vi "Remove_FF_lone_spikes.vi"(5 "Analysis Info cluster In":T1={"Colour"=0, "Inst type"=enum."Pitot-static tube", "Inst name"="Manometer voltage", "Symbol"="U", "Code name"="", "Extra Info"="U", "Inst Array"=enum."PWA", "U"=0.0, "u^2"=0.0, "u^3"=0.0, "u^4"=0.0, "Skew_u"=0.0, "Kurt_u"=0.0, "Sd Error in Mean"=0.0, "% u'/U"=0.0, "X"=0.0, "Y"=0.0, "Z"=0.0, "Timescale integral Estimate"=0.0, "Sd Error in Variance"=0.0, "Calib File"=path "", "Calib Constants"=[], "Output Position"=FALSE, "Stats"=enum."None", "Av Sampling Rate"=0.0, "Av No of Samples"=0.0, "Total Meas Time (s)"=0.0, "OrigChName"="", "Max value"=0.0, "Min value"=0.0, "Req Sample Rate Hz"=0.0, "Sync Delay Time (s)"=0.0, "Ch No"=0, "Device"="", "Use Latest Calib"=FALSE, "Port"="", "Metadata Ch Names"=[], "Metadata Ch Values"=[], "Label"="", "chState"=enum."Solo", "Point Drift"=0.0, "inputConfig"=""} {"Kurt_u" format="%_3g"; "u^4" format="%_3g"; "u^3" format="%_3g"; "Sd Error in Variance" format="%_3g"; "u^2" format="%_3g"; "Sd Error in Mean" format="%_3g"; "U" format="%_3g"; "Sync Delay Time (s)" format="%.4f"; "Total Meas Time (s)" format="%_5g"; "Skew_u" format="%_3g"; "% u'/U" format="%_3g"}, 6 "Average Sampling Rate":dbl, 7 "index of element":i32, 8 "Per Block Plug Ins":string[](array[string]), 9 "Time Trace":dbl[](array[numeric])) -> (3 "Filtered Time Trace":dbl[](array[numeric]), 4 "Analysis Info cluster Out":T1={"Colour"=0, "Inst type"=enum."Pitot-static tube", "Inst name"="Manometer voltage", "Symbol"="U", "Code name"="", "Extra Info"="U", "Inst Array"=enum."PWA", "U"=0.0, "u^2"=0.0, "u^3"=0.0, "u^4"=0.0, "Skew_u"=0.0, "Kurt_u"=0.0, "Sd Error in Mean"=0.0, "% u'/U"=0.0, "X"=0.0, "Y"=0.0, "Z"=0.0, "Timescale integral Estimate"=0.0, "Sd Error in Variance"=0.0, "Calib File"=path "", "Calib Constants"=[], "Output Position"=FALSE, "Stats"=enum."None", "Av Sampling Rate"=0.0, "Av No of Samples"=0.0, "Total Meas Time (s)"=0.0, "OrigChName"="", "Max value"=0.0, "Min value"=0.0, "Req Sample Rate Hz"=0.0, "Sync Delay Time (s)"=0.0, "Ch No"=0, "Device"="", "Use Latest Calib"=FALSE, "Port"="", "Metadata Ch Names"=[], "Metadata Ch Values"=[], "Label"="", "chState"=enum."Solo", "Point Drift"=0.0, "inputConfig"=""} {"Kurt_u" format="%_3g"; "u^4" format="%_3g"; "u^3" format="%_3g"; "Sd Error in Variance" format="%_3g"; "u^2" format="%_3g"; "Sd Error in Mean" format="%_3g"; "U" format="%_3g"; "Sync Delay Time (s)" format="%.4f"; "Total Meas Time (s)" format="%_5g"; "Skew_u" format="%_3g"; "% u'/U" format="%_3g"})   [LabVIEW 2022 SP3]
uses:
  Globals/Meas_global.vi
  Controls/Inst_type.ctl
  Controls/Instrument_Array.ctl
  Controls/Analysis_info_cluster.ctl
  Controls/channelState.ctl
panel:
  out "Spikes Array Out":cluster{"Index":i32, "max value":dbl}[](array[cluster])
  out "Spikes Removed this block":i32
  out "Time Trace":dbl[][](graph)
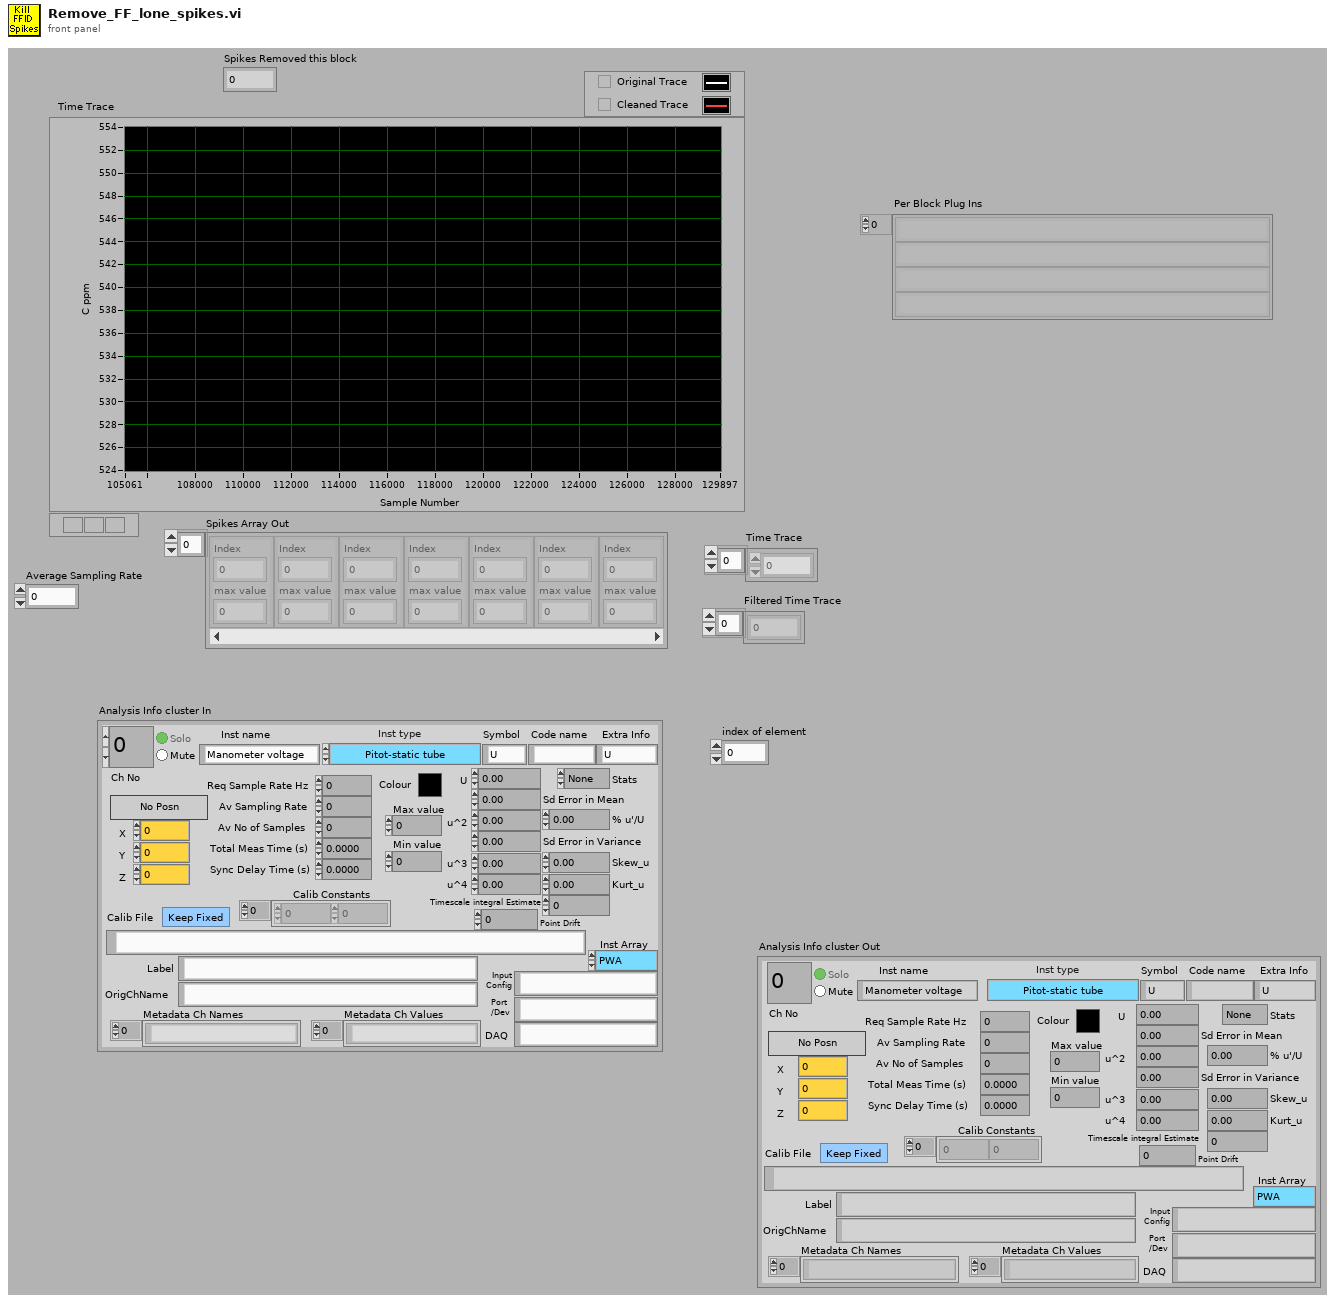
[diagram p1: front panel]
types:
  T1 = typedef "Analysis_info_cluster.ctl" = cluster{"Colour":u32, "Inst type":T2, "Inst name":string, "Symbol":string, "Code name":string, "Extra Info":string, "Inst Array":T3, "U":dbl, "u^2":dbl, "u^3":dbl, "u^4":dbl, "Skew_u":dbl, "Kurt_u":dbl, "Sd Error in Mean":dbl, "% u'/U":dbl, "X":dbl, "Y":dbl, "Z":dbl, "Timescale integral Estimate":dbl, "Sd Error in Variance":dbl, "Calib File":path, "Calib Constants":dbl[], "Output Position":bool, "Stats":enum16{"None", "Basic", "Full"}, "Av Sampling Rate":dbl, "Av No of Samples":dbl, "Total Meas Time (s)":dbl, "OrigChName":string, "Max value":dbl, "Min value":dbl, "Req Sample Rate Hz":dbl, "Sync Delay Time (s)":dbl, "Ch No":i16, "Device":string, "Use Latest Calib":bool, "Port":string, "Metadata Ch Names":string[], "Metadata Ch Values":string[], "Label":string, "chState":T4, "Point Drift":dbl, "inputConfig":string}
  T2 = typedef "Inst_type.ctl" = enum16{"Raw voltage", "Raw with zero offsetting", "Propeller anemometer", "Pressure Transducer", "Pitot-static tube", "Hot wire", "Cross wire 1", "Cross wire 2", "Generic Linear", "Generic Polynomial", "Generic BackPoly", "Fast FID", "Thermocouple", "Cold wire", "Pulsed Wire", "LDA Vel", "LDA Tran time", "LDA Arr time", "Microphone"}
  T3 = typedef "Instrument_Array.ctl" = enum16{"PWA", "LDA", "Analogue"}
  T4 = typedef "channelState.ctl" = enum32{"No Selection", "Solo", "Mute"}
  T5 = cluster{"Spikes Array Out":cluster{"Index":i32, "max value":dbl}[]}
  T6 = cluster{"Spikes Array Out":cluster{"Index":i32, "max value":dbl}[]}[]
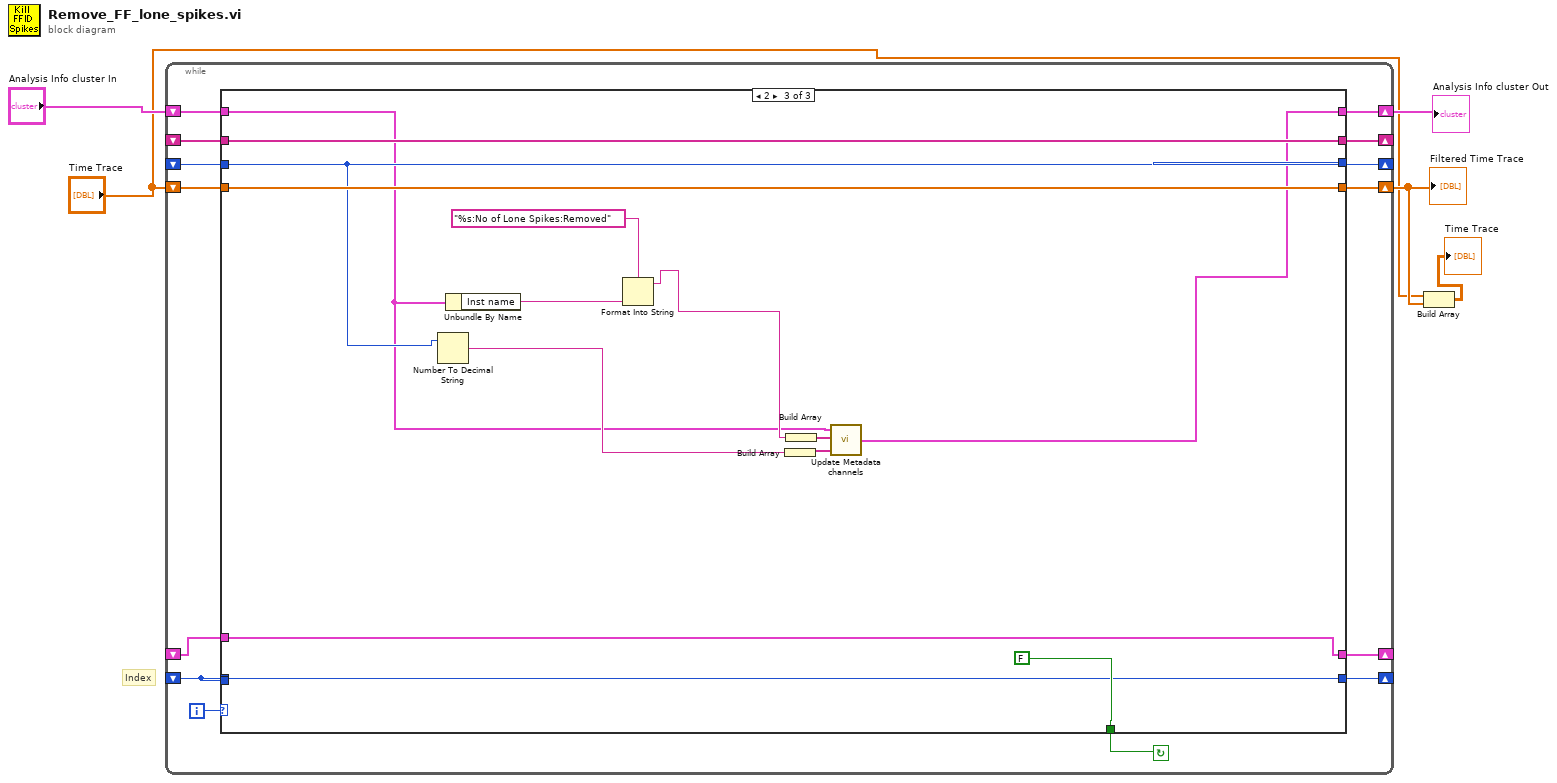
[diagram p0: block diagram]
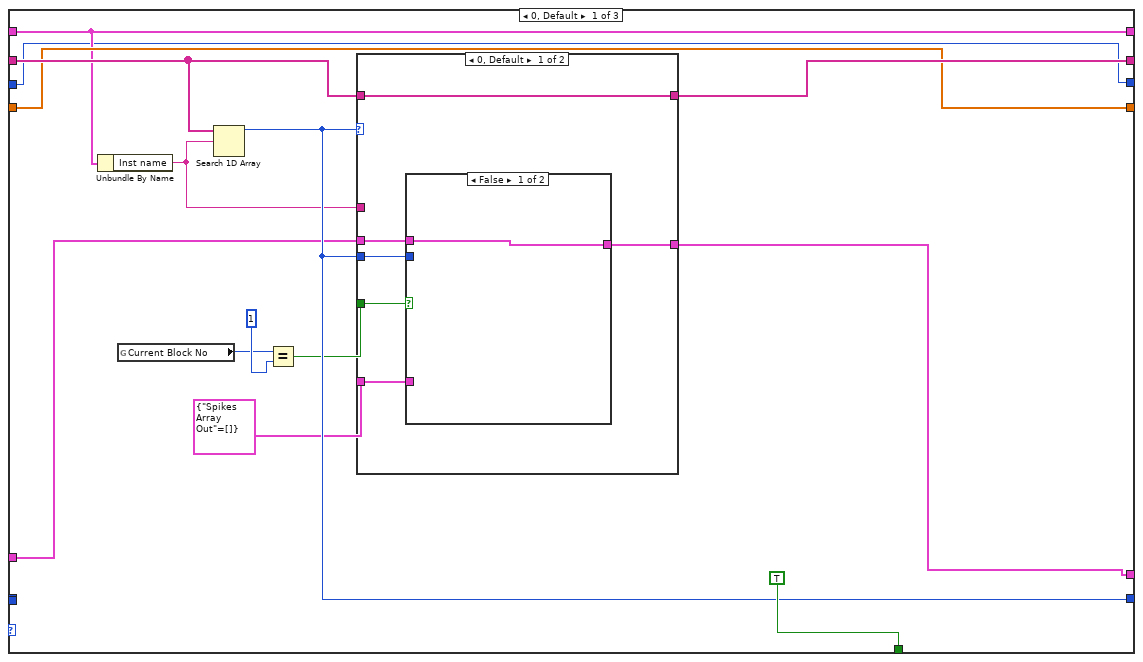
[diagram p2: hidden frame]
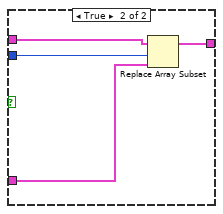
[diagram p3: hidden frame]
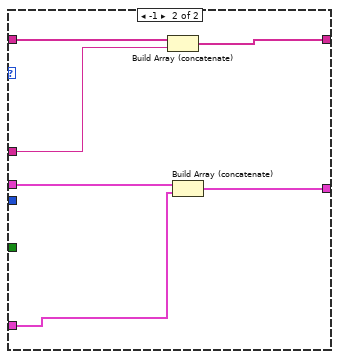
[diagram p4: hidden frame]
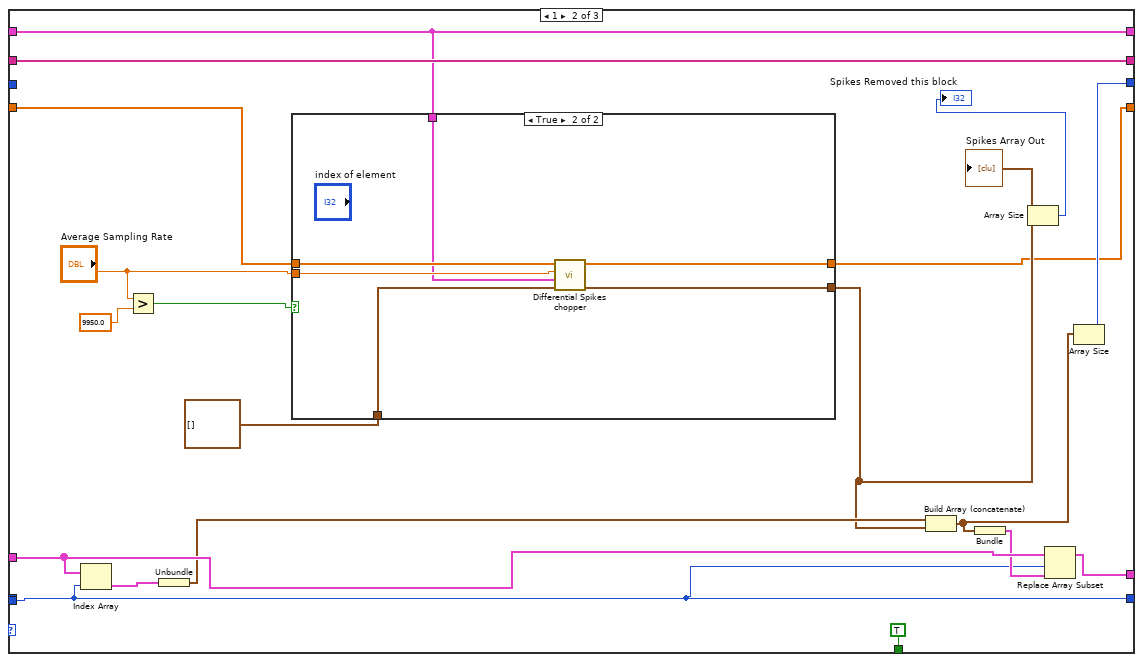
[diagram p5: hidden frame]
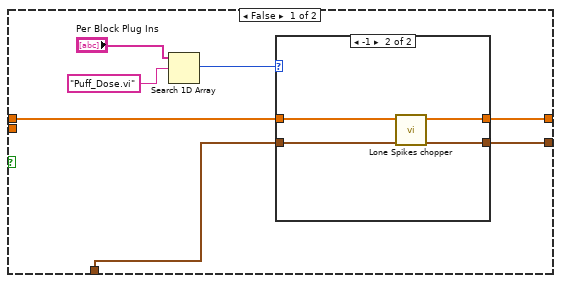
[diagram p6: hidden frame]
diagram:
  # "Index"
  n1 = while {
    shift-left: _ -> [w16]
    shift-right: [w18] -> _
    shift-right: [w14] -> _
    shift-left: _ -> [w15]
    shift-right: [w12] -> _
    shift-left: _ -> [w13]
    shift-right: [w10] -> w5
    shift-left: "Analysis Info cluster In" -> [w11]
    shift-right: [w8] -> w4
    shift-left: "Time Trace" -> [w9]
    shift-right: [w7] -> _
    shift-left: _ -> [w6]
    i -> [w19]
    stop <- w17 continue-if-true
    n2 = case shown="2" w19 {
      tunnel: [w28 w53 w101] -> w18
      tunnel: [TRUE TRUE ("Processing last block?") FALSE ("Processing last block?")] -> w17
      tunnel: w16 -> [_ _ w101]
      tunnel: w16 -> [_ w53 _]
      tunnel: w15 -> [w30 w69 w100]
      tunnel: [w29 w69 w100] -> w14
      tunnel: w13 -> [w20 _ w96]
      tunnel: [w20 w63 w96] -> w12
      tunnel: w11 -> [w25 w51 w90]
      tunnel: [w25 w51 w89] -> w10
      tunnel: w9 -> [w26 w59 w99]
      tunnel: [w26 w56 w99] -> w8
      tunnel: [w21 w66 w95] -> w7
      tunnel: w6 -> [w23 w67 w95]
      frame 0, Default {
        n3 = Unbundle By Name(w25) -> ("Inst name"=w24:string)
        n4 = global read "Meas_global.vi" "Current Block No"() -> (w32:i32)
        n5 = Search 1D Array(1D array=w30, element=w24) -> (index of element=w28:i32)  [unwired: 1 out]
        n6 = Equal?(x=w32, y=1) -> (x = y?=w27:bool)
        n7 = case shown="0, Default" w28 {
          tunnel: w30 -> [w39 w50]
          tunnel: w24 -> [_ w49]
          tunnel: [w39 w48] -> w29
          tunnel: w23 -> [w38 w47]
          tunnel: [w37 w46] -> w21
          tunnel: w28 -> [w36 _]
          tunnel: w27 -> [w35 _]
          tunnel: T5 {"Spikes Array Out"=[]} ("element") -> [w34 w45]
          frame 0, Default {
            n8 = case shown="False" w35 {
              tunnel: w38 -> [w40 w44]
              tunnel: [w40 w43] -> w37
              tunnel: w36 -> [_ w42]
              tunnel: w34 -> [_ w41]
              frame False {
              }
              frame True {
                n9 = Replace Array Subset(array=w44, new element=w41, index=w42) -> (w43:T6)
              }
            }
          }
          frame -1 {
            n10 = Build Array (concatenate)(w50, w49) -> (w48:string[])
            n11 = Build Array (concatenate)(w47, w45) -> (w46:T6)
          }
        }
      }
      frame 1 {
        n12 = Index Array(array=w67, index=w53) -> (element=w64:T5)
        n13 = Greater?(x="Average Sampling Rate", y=9950.0) -> (0:w54:bool)
        n14 = Unbundle(w64) -> ("Spikes Array Out"=w62:cluster{"Index":i32, "max value":dbl}[])
        n15 = case shown="True" w54 {
          tunnel: w59 -> [w76 w88]
          tunnel: cluster{"Index":i32, "max value":dbl}[] [] ("Spikes Array In") -> [w75 w87]
          tunnel: [w74 w83] -> w57
          tunnel: [w73 w84] -> w56
          tunnel: "Average Sampling Rate" -> [_ w86]
          tunnel: w51 -> [_ w85]
          frame False {
            n16 = Search 1D Array(1D array="Per Block Plug Ins", element="Puff_Dose.vi") -> (index of element=w70:i32)  [unwired: 1 in]
            n17 = case shown="-1" w70 {
              tunnel: w76 -> [w78 w82]
              tunnel: w75 -> [w77 w81]
              tunnel: [w77 w80] -> w74
              tunnel: [w78 w79] -> w73
              frame Default {
              }
              frame -1 {
                n18 = call "Lone Spikes chopper.vi"("Spikes Array In"=w81, "C Trace"=w82) -> ("Spikes Array Out"=w80:cluster{"Index":i32, "max value":dbl}[], "Filtered Time Trace"=w79:dbl[])  [unwired: 2 in, 2 out]
              }
            }
          }
          frame True {
            n19 = call "Differential Spikes chopper.vi"("Spikes Array In"=w87, "Analysis Info cluster In"=w85, "Average Sampling Rate"=w86, "C Trace"=w88) -> ("Spikes Array Out"=w83:cluster{"Index":i32, "max value":dbl}[], "Filtered Time Trace"=w84:dbl[])  [unwired: 1 in, 1 out]
          }
        }
        "Spikes Array Out" <- w57
        n20 = Build Array (concatenate)(w62, w57) -> (w61:cluster{"Index":i32, "max value":dbl}[])
        n21 = Bundle(w61) -> (w65:cluster{cluster{"Index":i32, "max value":dbl}[]})  [unwired: 1 in]
        n22 = Array Size(array=w57) -> (size(s)=→"Spikes Removed this block":i32)
        n23 = Replace Array Subset(array=w67, new element=w65, index=w53) -> (w66:T6)
        n24 = Array Size(array=w61) -> (size(s)=w63:i32)
      }
      frame 2 {
        n25 = Number To Decimal String(number=w96) -> (decimal integer string=w93:string)  [unwired: 1 out]
        n26 = Unbundle By Name(w90) -> ("Inst name"=w98:string)
        n27 = Format Into String(format string="%s:No of Lone Spikes:Removed", w98) -> (resulting string=w92:string)  [unwired: 2 in, 1 out]
        n28 = Build Array(w93) -> (w94:string[])
        n29 = Build Array(w92) -> (w91:string[])
        n30 = call "Update Metadata channels.vi"("Metadata Values"=w94, "Metadata Names"=w91, "Analysis info Cluster in"=w90) -> ("Analysis info Cluster out"=w89:T1)
      }
    }
  }
  "Filtered Time Trace" <- w4
  "Analysis Info cluster Out" <- w5
  n31 = Build Array("Time Trace", w4) -> (→"Time Trace":dbl[][])
